vi "MH-Dequeue Message.vi"(0 "MH Queue":refnum<queue>) -> (4 "MH Queue out":refnum<queue>, 6 "Message":string, 10 "Data":variant, 15 "error out":errorcluster)   [LabVIEW 2020]
uses:
  MH-Message.ctl
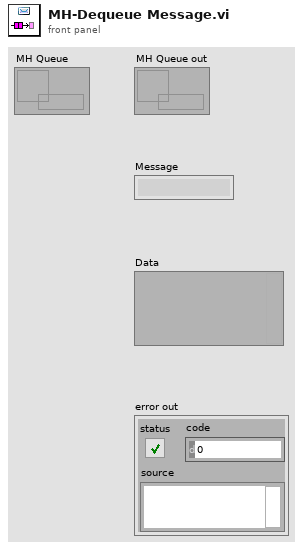
[diagram p1: front panel]
types:
  T1 = typedef "MH-Message.ctl" = cluster{"Message":string, "Data":variant}
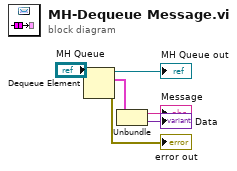
[diagram p0: block diagram]
diagram:
  n1 = Dequeue Element(queue="MH Queue") -> (queue out=→"MH Queue out":refnum<queue>, element=w3:T1, error out=→"error out":errorcluster)  [unwired: 2 in, 1 out]
  n2 = Unbundle(w3) -> ("Message"=→"Message":string, "Data"=→"Data":variant)
